vi "XY Graph Load Plot(s) from ASCII File.vi"(7 "Header Definitions":T2, 8 "error in (no error)":errorcluster, 10 "Delimiter (TAB)":string="\t", 11 "File Path":path) -> (0 "error out":errorcluster, 1 "Plot Scales Array":T1[](array[typedef]), 2 "Plot Name Array":string[](array[string]), 3 "Plot Array":cluster{"X Array":dbl[], "Y Array":dbl[]}[](array[cluster]), 4 "Time (s)":dbl)   [LabVIEW 2019, in "XY Graph Add-Ons.lvlib"]
uses:
  XY Graph Add-Ons.lvlib
  Files/ASCII File Header Definition.ctl
  Plot Scale Labels.ctl
  <vilib>/Utility/High Resolution Relative Seconds.vi
  <vilib>/Utility/error.llb/Error Cluster From Error Code.vi
  <vilib>/ErrorRing/Error Ring.xnode
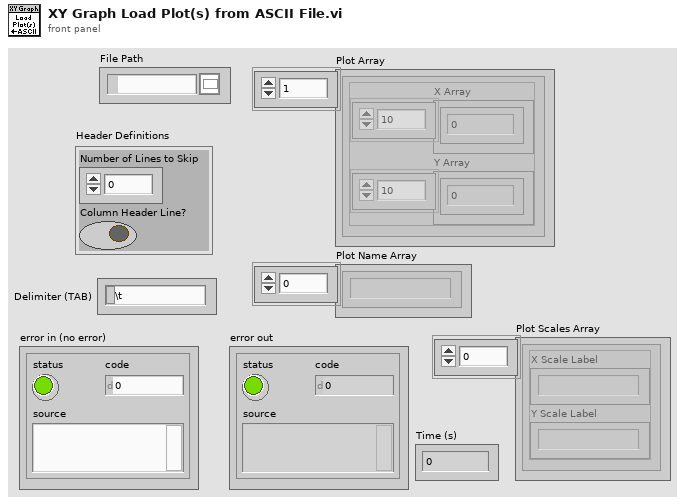
[diagram p1: front panel]
types:
  T1 = typedef "Plot Scale Labels.ctl" = cluster{"X Scale Label":string, "Y Scale Label":string}
  T2 = typedef "ASCII File Header Definition.ctl" = cluster{"Number of Lines to Skip":i32, "Column Header Line?":bool}
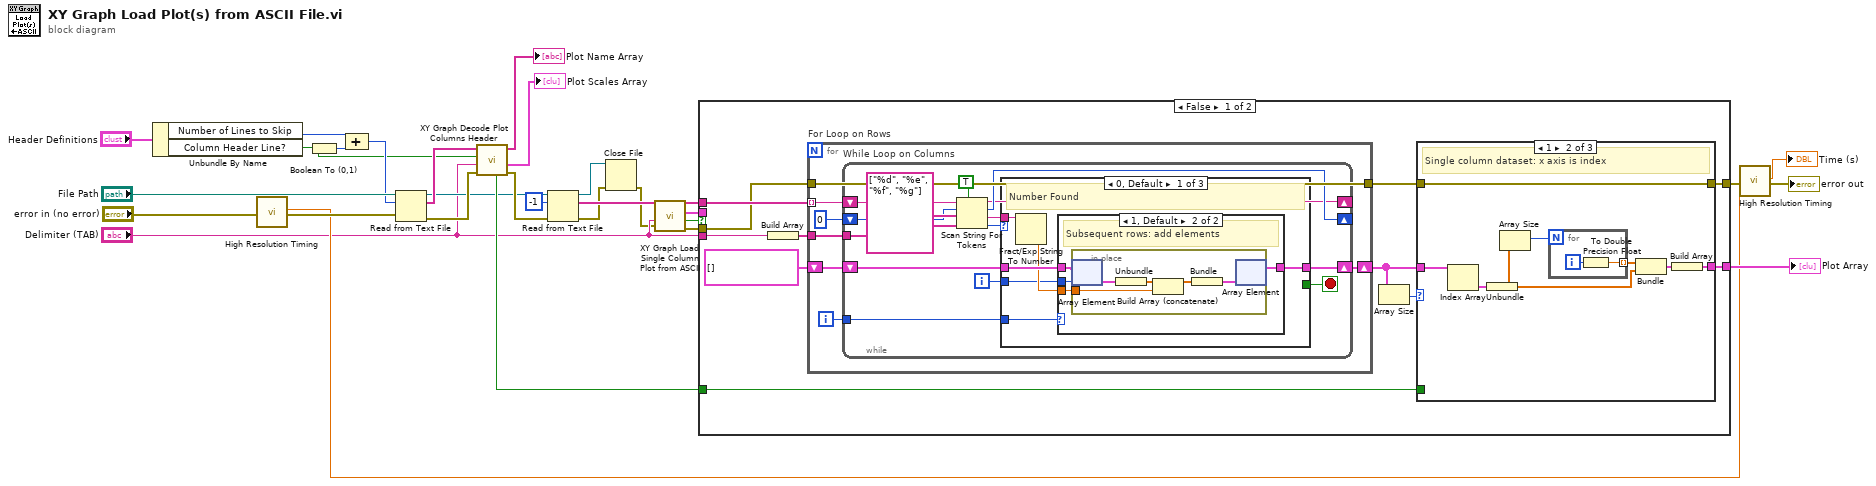
[diagram p0: block diagram]
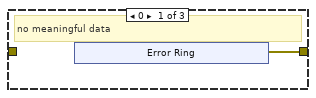
[diagram p2: hidden frame]
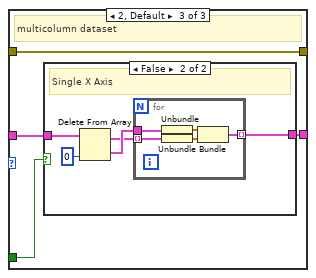
[diagram p3: hidden frame]
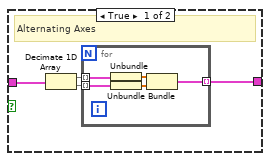
[diagram p4: hidden frame]
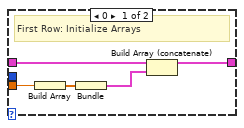
[diagram p5: hidden frame]
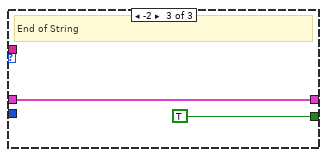
[diagram p7: hidden frame]
diagram:
  n1 = Unbundle By Name("Header Definitions") -> ("Number of Lines to Skip"=w28:i32, "Column Header Line?"=w21:bool)
  n2 = call "High Resolution Timing.vi"("Error In"="error in (no error)") -> ("elapsed (relative) seconds"=w14:dbl, "Error Out"=w17:errorcluster)  [unwired: 16 in, 1 out]
  n3 = Boolean To (0,1)(Boolean=w21) -> (0, 1=w27:i16)
  n4 = Compound Arithmetic op=ADD(w28, w27) -> (w26:i32)
  n5 = Read from Text File(file (use dialog)="File Path", count=w26, error in=w17) -> (refnum out=w9:refnum<file>, text=w24:string[], error out=w22:errorcluster)  [unwired: 1 in, 1 out]
  n6 = call "XY Graph Decode Plot Columns Header.vi"("Error In"=w22, "Delimiter"="Delimiter (TAB)", "Column Header Line? (F)"=w21, "Header String Array"=w24) -> ("Error Out"=w12:errorcluster, "Plot Scales Array"=→"Plot Scales Array":T1[], "Plot Name Array"=→"Plot Name Array":string[], "Alternating Axes?"=w18:bool)  [unwired: 4 in]
  n7 = Read from Text File(file (use dialog)=w9, count=-1, error in=w12) -> (refnum out=w10:refnum<file>, text=w8:string[], error out=w3:errorcluster)  [unwired: 1 in, 1 out]
  n8 = Close File(refnum=w10, error in=w3) -> (error out=w2:errorcluster)  [unwired: 1 out]
  n9 = call "XY Graph Load Single Column Plot from ASCII.vi"("error in (no error)"=w2, "Delimiter (TAB)"="Delimiter (TAB)", "String Array"=w8) -> ("error out"=w7:errorcluster, "Single Column?"=w6:bool, "Plot Array"=w5:cluster{"Array":dbl[], "Array":dbl[]}[], "String Array dup"=w1:string[])  [unwired: 5 in]
  n10 = case shown="False" w6 {
    tunnel: [w41 w125] -> w23
    tunnel: w18 -> [w40 _]
    tunnel: [w39 w124] -> w16
    tunnel: w1 -> [w33 _]
    tunnel: "Delimiter (TAB)" -> [w32 _]
    tunnel: w7 -> [w31 w124]
    tunnel: w5 -> [_ w125]
    frame False {
      n11 = Build Array(w32) -> (w38:string[])
      n12 = for "For Loop on Rows" {
        tunnel: w33 -> [w86] mode=indexing
        tunnel: w38 -> [w85]
        shift-right: [w82] -> w36
        shift-left: cluster{dbl[]}[] [] -> [w83]
        tunnel: w31 -> [w80]
        tunnel: [w80] -> w34
        i -> [w81]
        n13 = while "While Loop on Columns" {
          tunnel: w85 -> [w99]
          shift-right: [w95] -> _
          shift-left: w86 -> [w100]
          shift-right: [w96] -> _
          shift-left: 0 ("offset past token") -> [w97]
          shift-right: [w89] -> w82
          shift-left: w83 -> [w91]
          tunnel: w81 -> [w88]
          i -> [w90]
          stop <- w92 stop-if-true
          n14 = Scan String For Tokens(5:TRUE ("allow empty tokens? (F)"), 6:w99, 7:string[] ["%d", "%e", "%f", "%g"] ("operators (none)"), 8:w97, 9:w100) -> (0:w94:i32, 1:w93:string, 2:w96:i32, 3:w95:string)  [unwired: 1 in]
          n15 = case shown="0, Default" w94 {
            tunnel: w93 -> [w106 _ _]
            tunnel: [_ _ TRUE] -> w92
            tunnel: w91 -> [w105 w121 w122]
            tunnel: w90 -> [w102 _ _]
            tunnel: [w103 w121 w122] -> w89
            tunnel: w88 -> [w101 _ _]
            frame 0, Default {
              # "Number Found"
              n16 = Fract/Exp String To Number(string=w106) -> (number=w104:dbl)  [unwired: 3 in, 1 out]
              n17 = case shown="1, Default" w101 {
                tunnel: w105 -> [w109 w115]
                tunnel: w104 -> [w111 w114]
                tunnel: [w107 w113] -> w103
                tunnel: w102 -> [_ w112]
                frame 0 {
                  # "First Row: Initialize Arrays"
                  n18 = Build Array(w111) -> (w110:dbl[])
                  n19 = Bundle(w110) -> (w108:cluster{dbl[]})  [unwired: 1 in]
                  n20 = Build Array (concatenate)(w109, w108) -> (w107:cluster{dbl[]}[])
                }
                frame 1, Default {
                  # "Subsequent rows: add elements"
                  n21 = in-place {
                    in-place-border: w114 -> [w119]
                    n22 = in-place-array #1(w115, w112) -> (w120:cluster{dbl[]})
                    n23 = Unbundle(w120) -> (w117:dbl[])
                    n24 = Build Array (concatenate)(w117, w119) -> (w118:dbl[])
                    n25 = Bundle(w118) -> (w116:cluster{dbl[]})  [unwired: 1 in]
                    n26 = in-place-array #1(w116) -> (w113:cluster{dbl[]}[])  [unwired: 1 out]
                  }
                }
              }
            }
            frame -1 {
              # "Some columns have less numbers than others"
              # "Number not Found"
            }
            frame -2 {
              # "End of String"
            }
          }
        }
      }
      n27 = Array Size(array=w36) -> (size(s)=w35:i32)
      n28 = case shown="1" w35 {
        tunnel: [_ w48 w60] -> w41
        tunnel: w40 -> [_ _ w59]
        tunnel: w36 -> [_ w54 w58]
        tunnel: w34 -> [_ w47 w57]
        tunnel: [w42 w47 w57] -> w39
        frame 0 {
          # "no meaningful data"
          n29 = xnode "Error Ring"() -> ("error out"=w42:errorcluster)
        }
        frame 1 {
          # "Single column dataset: x axis is index"
          n30 = Index Array(array=w54) -> (element=w53:cluster{dbl[]})  [unwired: 1 in]
          n31 = Unbundle(w53) -> (w50:dbl[])
          n32 = Array Size(array=w50) -> (size(s)=w52:i32)
          n33 = for {
            N: w52 -> [_]
            tunnel: [w55] -> w51 mode=indexing
            i -> [w56]
            n34 = To Double Precision Float(number=w56) -> (double precision float=w55:dbl)
          }
          n35 = Bundle(w51, w50) -> (w49:cluster{dbl[], dbl[]})  [unwired: 1 in]
          n36 = Build Array(w49) -> (w48:cluster{dbl[], dbl[]}[])
        }
        frame 2, Default {
          # "multicolumn dataset"
          n37 = case shown="False" w59 {
            tunnel: w58 -> [w64 w73]
            tunnel: [w61 w74] -> w60
            frame True {
              # "Alternating Axes"
              n38 = Decimate 1D Array(w64) -> (w63:cluster{dbl[]}[], w62:cluster{dbl[]}[])
              n39 = for {
                tunnel: w63 -> [w69] mode=indexing
                tunnel: w62 -> [w68] mode=indexing
                tunnel: [w65] -> w61 mode=indexing
                n40 = Unbundle(w69) -> (w67:dbl[])
                n41 = Unbundle(w68) -> (w66:dbl[])
                n42 = Bundle(w67, w66) -> (w65:cluster{dbl[], dbl[]})  [unwired: 1 in]
              }
            }
            frame False {
              # "Single X Axis"
              n43 = Delete From Array(array=w73, index=0) -> (deleted portion=w71:cluster{dbl[]}, array with subset deleted=w70:cluster{dbl[]}[])  [unwired: 1 in]
              n44 = for {
                tunnel: w71 -> [w79]
                tunnel: w70 -> [w78] mode=indexing
                tunnel: [w75] -> w74 mode=indexing
                n45 = Unbundle(w79) -> (w77:dbl[])
                n46 = Unbundle(w78) -> (w76:dbl[])
                n47 = Bundle(w77, w76) -> (w75:cluster{dbl[], dbl[]})  [unwired: 1 in]
              }
            }
          }
        }
      }
    }
    frame True {
    }
  }
  "Plot Array" <- w23
  n48 = call "High Resolution Timing.vi"("relative seconds (NaN)"=w14, "Error In"=w16) -> ("elapsed (relative) seconds"=→"Time (s)":dbl, "Error Out"=→"error out":errorcluster)  [unwired: 15 in, 1 out]
